vi "CD Init Incoming Single Point Signals.vi"(8 "error in":errorcluster, 9 "database":T1, 10 "can port":string, 11 "XNET Cluster":refnum<k21>) -> (0 "error out":errorcluster, 1 "Incoming Single Point Configuraiton":T5, 2 "initial value":dbl[](array[numeric]), 3 "channels":refnum<class "TBM channel.lvclass">[](array[class]), 4 "# of Channels":u32, 5 "inputs":T4[](array[typedef]), 7 "input IDs":string[](array[string]))   [LabVIEW 2013, in "J1939.lvlib"]
uses:
  J1939.lvlib
  CD Incoming Single Point Configuration.ctl
  CD Incoming Single Point Frame Pairs.ctl
  API Types/Signal Mapping.ctl
  <vilib>/NI/Tag Bus/tag/Data Type.ctl
  <vilib>/NI/Tag Bus Module Framework/channel/TBM channel.lvclass
  CD Conversion Lookup Table Parameters Cluster.ctl
  Configuration/TypeDefs/J1939 db.ctl
  Configuration/TypeDefs/J1939 db frame.ctl
  Configuration/TypeDefs/J1939 db signal.ctl
  Configuration/TypeDefs/J1939 db frame direction.ctl
  <vilib>/NI/Tag Bus Module Framework/channel/channel classification.ctl
  <vilib>/NI/Tag Bus/tag/tag descriptor.lvclass/tag descriptor.ctl
  Frame Conversion/Common Conversions.vi
  Frame Conversion/Convert CAN Arb ID to J1939 ID.vi
  <vilib>/xnet/xnet.llb/XNET Create Session (Conversion).vi
  <resource>/objmgr/xnet.rc
  <vilib>/NI/Tag Bus/tag/tag descriptor.lvclass
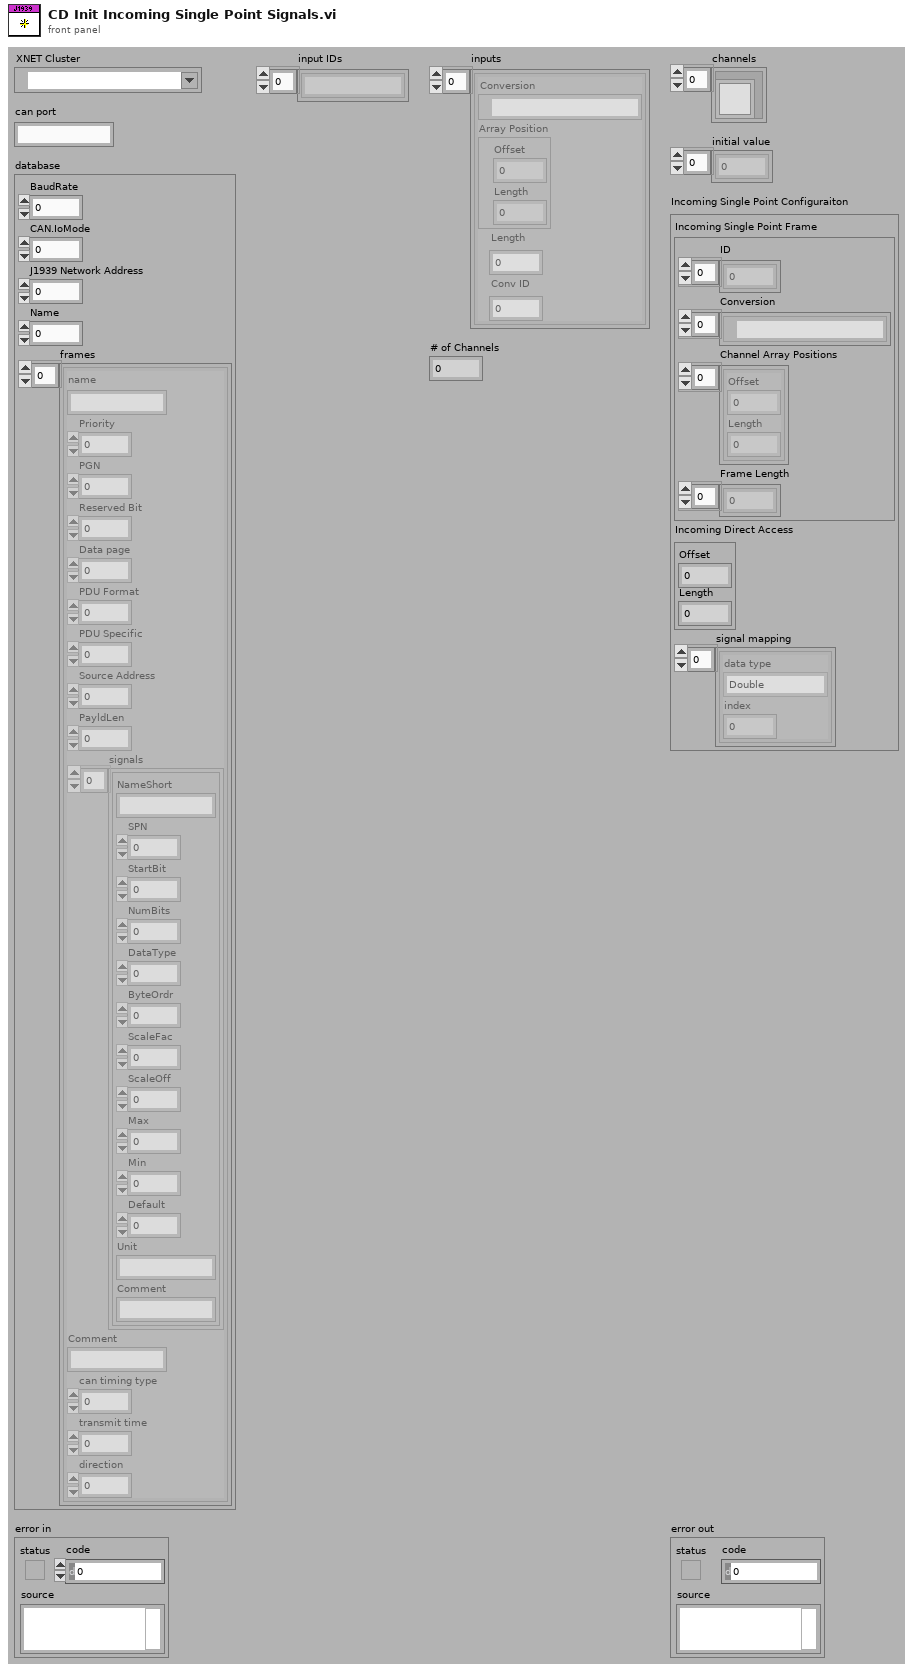
[diagram p1: front panel]
types:
  T1 = typedef "J1939.lvlib/J1939 db.ctl" = cluster{"BaudRate":u32, "CAN.IoMode":u32, "J1939 Network Address":u8, "Name":u64, "frames":T2[]}
  T2 = typedef "J1939.lvlib/J1939 db frame.ctl" = cluster{"name":string, "Priority":u8, "PGN":u32, "Reserved Bit":u8, "Data page":u8, "PDU Format":u8, "PDU Specific":u8, "Source Address":u8, "PayldLen":u32, "signals":T3[], "Comment":string, "can timing type":u32, "transmit time":dbl, "direction":u16}
  T3 = typedef "J1939.lvlib/J1939 db signal.ctl" = cluster{"NameShort":string, "SPN":i32, "StartBit":u32, "NumBits":u32, "DataType":u32, "ByteOrdr":u32, "ScaleFac":dbl, "ScaleOff":dbl, "Max":dbl, "Min":dbl, "Default":dbl, "Unit":string, "Comment":string}
  T4 = typedef "J1939.lvlib/CD Conversion Lookup Table Parameters Cluster.ctl" = cluster{"Conversion":refnum<k21>, "Array Position":cluster{"Offset":u32, "Length":u32}, "Length":u32, "Conv ID":u32}
  T5 = typedef "J1939.lvlib/CD Incoming Single Point Configuration.ctl" = cluster{"Incoming Single Point Frame":T6, "Incoming Direct Access":cluster{"Offset":u32, "Length":u32}, "signal mapping":T7[]}
  T6 = typedef "J1939.lvlib/CD Incoming Single Point Frame Pairs.ctl" = cluster{"ID":u32[], "Conversion":refnum<k21>[], "Channel Array Positions":cluster{"Offset":u32, "Length":u32}[], "Frame Length":u32[]}
  T7 = typedef "J1939.lvlib/signal mapping.ctl" = cluster{"data type":T8, "index":i32}
  T8 = typedef "tag bus.lvlib/tag descriptor.lvclass/Data Type.ctl" = enum16{"Double", "Single", "I64", "I32", "I16", "I8", "U64", "U32", "U16", "U8", "Boolean", "String", "Array of Double", "Array of Single", "Array of I64", "Array of I32", "Array of I16", "Array of I8", "Array of U64", "Array of U32", "Array of U16", "Array of U8", "Array of Boolean", "Array of String"}
  T9 = typedef "J1939.lvlib/J1939 db frame direction.ctl" = enum16{"Input", "Output", "Input+Output"}
  T10 = typedef "TBM channel.lvclass/channel classification.ctl" = enum16{"input data", "output data", "processing parameter", "processing result"}
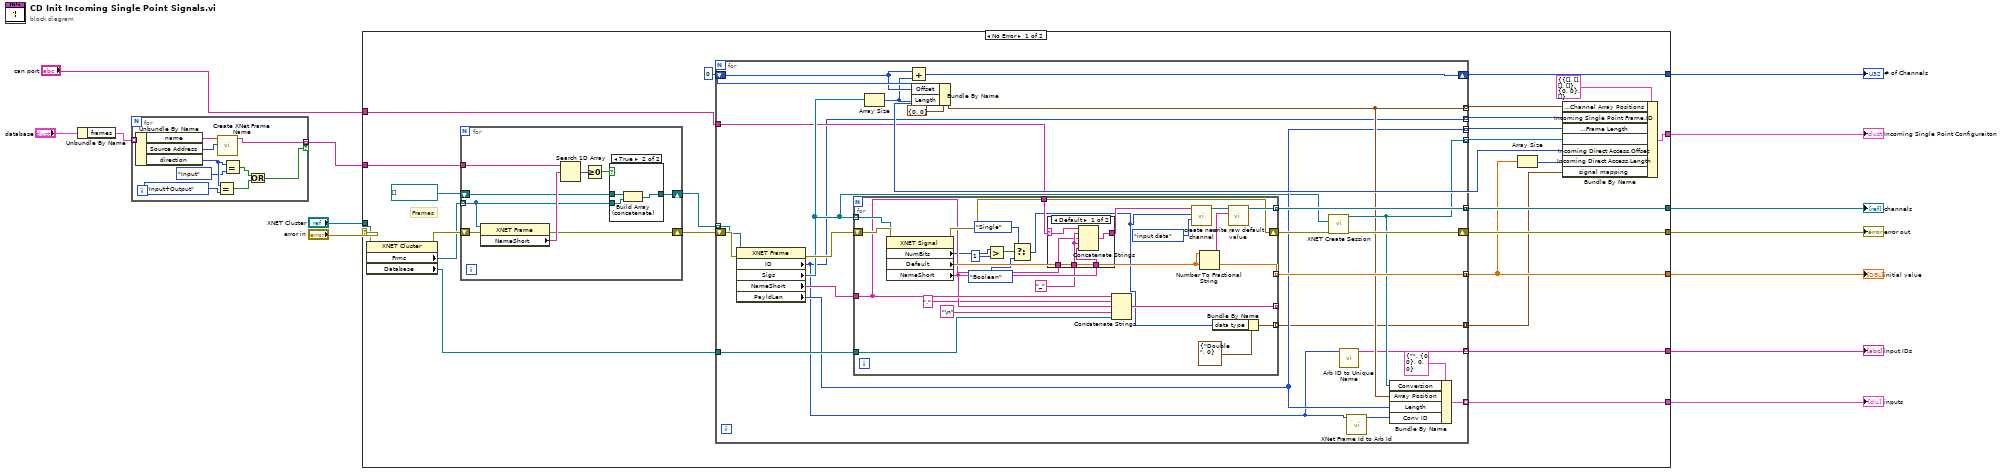
[diagram p0: block diagram]
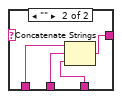
[diagram p3: hidden frame]
diagram:
  n1 = Unbundle By Name("database") -> ("frames"=w2:T2[])
  n2 = for {
    tunnel: w2 -> [w23] mode=indexing
    tunnel: [w20] -> w1 mode=indexing if=w14
    n3 = Unbundle By Name(w23) -> ("name"=w22:string, "Source Address"=w21:u8, "direction"=w19:u16)
    n4 = Equal?(x=w19, y=J1939_db_frame_direction."Input+Output" ("Direction")) -> (x = y?=w16:bool)
    n5 = call "Create XNet Frame Name.vi"("Source Address"=w21, "name"=w22) -> ("String"=w20:string)  [unwired: 8 in, 1 out]
    n6 = Equal?(x=w19, y=J1939_db_frame_direction."Input" ("Direction")) -> (x = y?=w15:bool)
    n7 = Or(x=w15, y=w16) -> (x .or. y?=w14:bool)
  }
  n8 = case shown="No Error" "error in" {
    selector: "error in" -> [w41 w120]
    tunnel: [w47 _] -> w11
    tunnel: [w42 w120] -> w13
    tunnel: [w35 _] -> w10
    tunnel: [w34 _] -> w9
    tunnel: [w33 _] -> w8
    tunnel: [w32 _] -> w7
    tunnel: [w30 _] -> w6
    tunnel: "XNET Cluster" -> [w26 _]
    tunnel: "can port" -> [w25 _]
    tunnel: w1 -> [w24 _]
    frame No Error {
      w31 = u32 0
      # "Frames"
      n9 = property class="XNET Cluster"(reference=w26, error in=w41) -> (error out=w39:errorcluster, "Frms"=w38:refnum<k21>[], "Database"=w27:refnum<k21>)  [unwired: 1 out]
      n10 = for {
        tunnel: w38 -> [w53] mode=indexing
        tunnel: w24 -> [w57]
        shift-right: [w52] -> w37
        shift-left: refnum<k21>[] [] -> [w49]
        shift-right: [w50] -> w36
        shift-left: w39 -> [w51]
        n11 = property class="XNET Frame"(reference=w53, error in=w51) -> (error out=w50:errorcluster, "NameShort"=w56:string)  [unwired: 1 out]
        n12 = Search 1D Array(1D array=w57, element=w56) -> (index of element=w55:i32)  [unwired: 1 in]
        n13 = Greater Or Equal To 0?(x=w55) -> (x >= 0?=w54:bool)
        n14 = case shown="True" w54 {
          tunnel: w49 -> [w58 w61]
          tunnel: w53 -> [_ w60]
          tunnel: [w58 w59] -> w52
          frame False {
          }
          frame True {
            n15 = Build Array (concatenate)(w61, w60) -> (w59:refnum<k21>[])
          }
        }
      }
      n16 = for {
        shift-right: [w85] -> w42
        shift-left: w36 -> [w80]
        tunnel: [w70] -> w45 mode=indexing
        tunnel: [w62] -> w46 mode=indexing
        shift-right: [w84] -> w35
        shift-left: w31 -> [w82]
        tunnel: [w69] -> w44 mode=indexing
        tunnel: [w68] -> w43 mode=indexing
        tunnel: w37 -> [w79] mode=indexing
        tunnel: w27 -> [w75]
        tunnel: [w74] -> w34 mode=concatenating
        tunnel: [w73] -> w30 mode=concatenating
        tunnel: [w71] -> w33 mode=indexing
        tunnel: [w67] -> w32 mode=indexing
        tunnel: [w66] -> w28 mode=concatenating
        tunnel: w25 -> [w64]
        n17 = property class="XNET Frame"(reference=w79, error in=w80) -> (error out=w77:errorcluster, "ID"=w62:u32, "Sigs"=w65:refnum<k21>[], "NameShort"=w78:string, "PayldLen"=w68:u32)  [unwired: 1 out]
        n18 = for {
          shift-right: [w103] -> w76
          shift-left: w77 -> [w110]
          tunnel: w65 -> [w98] mode=indexing
          tunnel: [w105] -> _ mode=indexing
          tunnel: w78 -> [w97]
          tunnel: w75 -> [w108]
          tunnel: [w102] -> w73 mode=indexing
          tunnel: [w104] -> w74 mode=indexing
          tunnel: [w99] -> w66 mode=indexing
          tunnel: w64 -> [w94]
          n19 = property class="XNET Signal"(reference=w98, error in=w110) -> (error out=w103:errorcluster, "NumBits"=w93:u32, "Default"=w102:dbl, "NameShort"=w96:string)  [unwired: 1 out]
          n20 = Greater?(x=w93, y=u32 1) -> (0:w91:bool)
          n21 = Select(t=Data_Type."Single" ("data type"), s=w91, f=Data_Type."Boolean" ("data type")) -> (s? t:f=w88:T8)
          n22 = case shown="Default" w94 {
            selector: w94 -> [w114 _]
            tunnel: w97 -> [w112 w119]
            tunnel: w96 -> [w111 w118]
            tunnel: "_" ("string") -> [w115 w117]
            tunnel: [w113 w116] -> w95
            frame Default {
              n23 = Concatenate Strings(w114, w115, w112, w115, w111) -> (w113:string)
            }
            frame "" {
              n24 = Concatenate Strings(w119, w117, w118) -> (w116:string)
            }
          }
          n25 = Concatenate Strings(w97, "." ("string"), w96, "\n" ("string"), w108) -> (w105:string)
          n26 = call <vilib>:"create new channel.vi"("channel classification"=channel_classification."input data", "data type"=w88, "channel name"=w95) -> ("channel"=w107:refnum<class "TBM channel.lvclass">)  [unwired: 8 in]
          n27 = Number To Fractional String(number=w102) -> (F-format string=w101:string)  [unwired: 3 in]
          n28 = Bundle By Name(cluster=T7 {"data type"=enum."Double", "index"=0}, "data type"=w88) -> (w99:T7)
          n29 = call <vilib>:"write raw default value.vi"("raw default"=w101, "system tag in"=w107) -> ("system tag out"=w104:refnum<class "TBM channel.lvclass">)  [unwired: 8 in, 1 out]
        }
        n30 = Array Size(array=w65) -> (size(s)=w81:i32)
        n31 = Add(x=w82, y=w81) -> (x+y=w84:u32)
        n32 = Bundle By Name(cluster=cluster{"Offset":u32, "Length":u32} {"Offset"=0, "Length"=0} ("Channel Array Position"), "Offset"=w82, "Length"=w81) -> (w69:cluster{"Offset":u32, "Length":u32})
        n33 = call-poly <vilib>:"XNET Create Session.vi"("signal list"=w65, "error in (no error)"=w76) -> ("session out"=w70:refnum<k21>, "error out"=w85:errorcluster)  [unwired: 12 in]
        n34 = call "Arb ID to Unique Name.vi"("Arb ID"=w62) -> ("name"=w67:string)  [unwired: 10 in]
        n35 = call "XNet Frame Id to Arb Id.vi"("ID"=w62) -> ("Arb id"=w63:u32)  [unwired: 10 in]
        n36 = Bundle By Name(cluster=T4 {"Conversion"="", "Array Position"={"Offset"=0, "Length"=0}, "Length"=0, "Conv ID"=0}, "Conversion"=w70, "Array Position"=w69, "Length"=w68, "Conv ID"=w63) -> (w71:T4)
      }
      n37 = Array Size(array=w30) -> (size(s)=w29:i32)
      n38 = Bundle By Name(cluster=T5 {"Incoming Single Point Frame"={"ID"=[], "Conversion"=[], "Channel Array Positions"=[], "Frame Length"=[]}, "Incoming Direct Access"={"Offset"=0, "Length"=0}, "signal mapping"=[]} ("Incoming Single Point Configuraiton"), "Incoming Single Point Frame.Channel Array Positions"=w44, "Incoming Single Point Frame.ID"=w46, "Incoming Single Point Frame.Frame Length"=w43, "Incoming Single Point Frame.Conversion"=w45, "Incoming Direct Access.Offset"=w31, "Incoming Direct Access.Length"=w29, "signal mapping"=w28) -> (w47:T5)
    }
    frame Error {
    }
  }
  "error out" <- w13
  "Incoming Single Point Configuraiton" <- w11
  "# of Channels" <- w10
  "channels" <- w9
  "input IDs" <- w7
  "inputs" <- w8
  "initial value" <- w6
